vi "Get Client URI.vi"(8 "error in (no error)":errorcluster, 11 "Request in":refnum<class "Request.lvclass">) -> (0 "error out":errorcluster, 2 "Client URI":refnum<class "URI.lvclass">, 3 "Request out":refnum<class "Request.lvclass">)   [LabVIEW 2020, in "HTTP Utils.lvlib" / "Request.lvclass"]
uses:
  Request.lvclass
  lv-uri/URI/URI/URI.lvclass
  Request.lvclass/Request.ctl
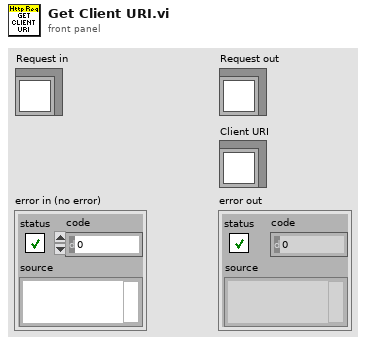
[diagram p1: front panel]
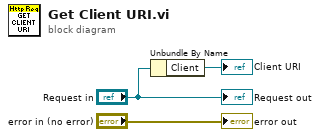
[diagram p0: block diagram]
diagram:
  n1 = Unbundle By Name("Request in") -> ("Client"=→"Client URI":refnum<class "URI.lvclass">)
  "error out" <- "error in (no error)"
  "Request out" <- "Request in"
